vi "INFOdll.vi"(8 "error in (no error)":errorcluster, 11 "icomp":i32) -> (0 "error out":errorcluster, 3 "INFO_OUT":T1)   [LabVIEW 2021]
doc: "subroutine INFO (icomp,wmm,ttrp,tnbpt,tc,pc,Dc,Zc,acf,dip,Rgas)\n\nProvides fluid constants for specified component\n\nINPUTS:\nicomp--component number in mixture; 1 for pure fluid\n\nOUTPUTS:\nwmm--molecular weight [g/mol]\nttrp--triple point temperature [K]\ntnbpt--normal boiling point temperature [K]\ntc--critical temperature [K]\npc--critical pressure [kPa]\nDc--critical density [mol/L]\nZc--compressibility at critical point [pc/(Rgas*Tc*Dc)]\nacf--acentric factor [-]\ndip--dipole moment [debye]\nRgas--gas constant [J/mol-K]"
uses:
  REFPROP.dll
panel:
  # "REFPROP-INFOdll.vi"
  # "void  INFOdll(int32_t *icomp, double *wmm, double *ttrp, double *tnbpt, double *tc, double *pc, double *dc, double *Zc, double *acf, double *dip, double *Rgas);"
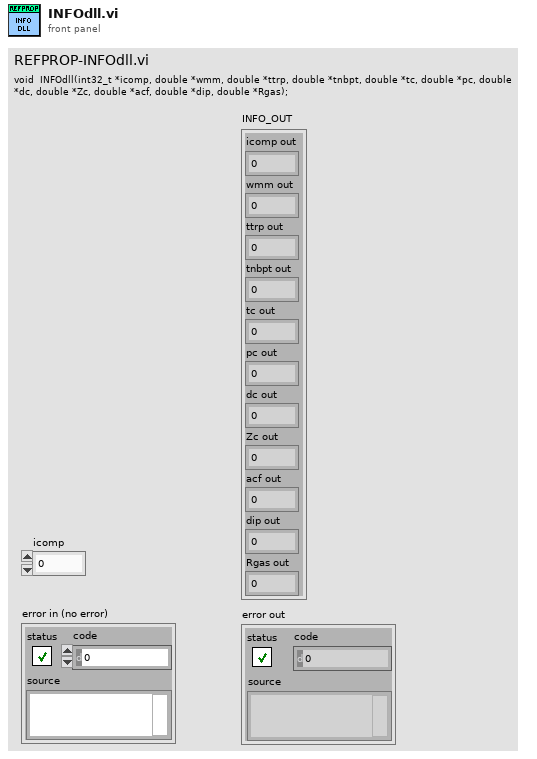
[diagram p1: front panel]
types:
  T1 = cluster{"icomp out":i32, "wmm out":dbl, "ttrp out":dbl, "tnbpt out":dbl, "tc out":dbl, "pc out":dbl, "dc out":dbl, "Zc out":dbl, "acf out":dbl, "dip out":dbl, "Rgas out":dbl}
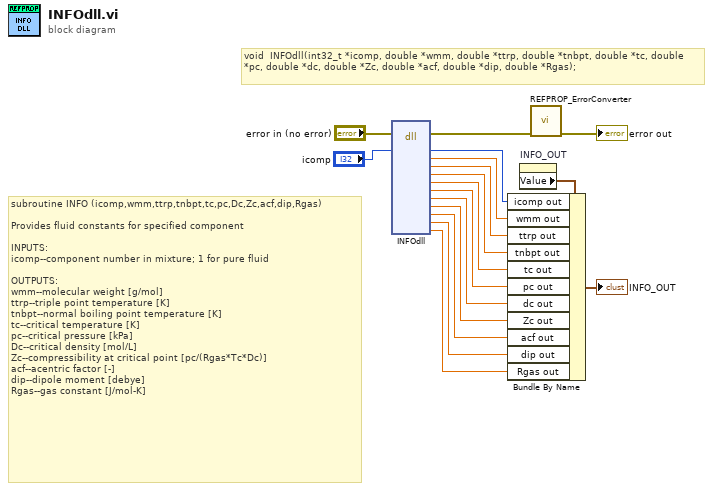
[diagram p0: block diagram]
diagram:
  # "void  INFOdll(int32_t *icomp, double *wmm, double *ttrp, double *tnbpt, double *tc, double *pc, double *dc, double *Zc, double *acf, double *dip, double *Rgas);"
  # "subroutine INFO (icomp,wmm,ttrp,tnbpt,tc,pc,Dc,Zc,acf,dip,Rgas)\n\nProvides fluid constants for specified component\n\nINPUTS:\nicomp--component number in mixture; 1 for pure fluid\n\nOUTPUTS:\nwmm--molecular weight [g/mol]\nttrp--triple point temperature [K]\ntnbpt--normal boiling point temperature [K]\ntc--critical temperature [K]\npc--critical pressure [kPa]\nDc--critical density [mol/L]\nZc--compressibility at critical point [pc/(Rgas*Tc*Dc)]\nacf--acentric factor [-]\ndip--dipole moment [debye]\nRgas--gas constant [J/mol-K]"
  n1 = dll-call lib="C:/Users/lauria/OneDrive - National Institute of Standards and Technology (NIST)/LabVIEW Projects/7 REFPROP/REFPROP-wrappers-master/REFPROP-wrappers-master/wrappers/Labview/REFPROP/REFPROP.*" fn="INFOdll"(error in="error in (no error)", "icomp"="icomp") -> (error out=w17:errorcluster, "icomp"=w14:i32, "wmm"=w4:dbl, "ttrp"=w3:dbl, "tnbpt"=w13:dbl, "tc"=w5:dbl, "pc"=w12:dbl, "dc"=w11:dbl, "Zc"=w10:dbl, "acf"=w9:dbl, "dip"=w7:dbl, "Rgas"=w6:dbl)  [unwired: 13 in, 1 out]
  n2 = property on="INFO_OUT" class="Clust (strict)"() -> ("Value"=w15:T1)  [unwired: 2 in, 2 out]
  n3 = Bundle By Name(cluster=w15, "icomp out"=w14, "wmm out"=w4, "ttrp out"=w3, "tnbpt out"=w13, "tc out"=w5, "pc out"=w12, "dc out"=w11, "Zc out"=w10, "acf out"=w9, "dip out"=w7, "Rgas out"=w6) -> (→"INFO_OUT":T1)
  n4 = call "REFPROP_ErrorConverter.vi"("error in (no error)"=w17) -> ("error out"=→"error out":errorcluster)  [unwired: 10 in]
